vi "ICM aI8.vi"(11 "String In":string) -> (1 "Value I8":i8, 2 "Value":dbl, 3 "String Out":string)   [LabVIEW 2018]
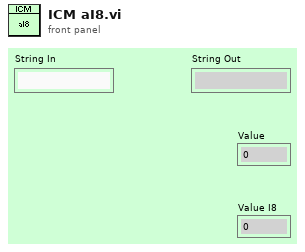
[diagram p1: front panel]
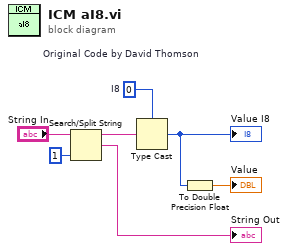
[diagram p0: block diagram]
diagram:
  w5 = i8 0  # I8
  n1 = Search/Split String(string="String In", offset (0)=1) -> (substring before match=w1:string, match + rest of string=→"String Out":string)  [unwired: 2 out]
  n2 = Type Cast "Original Code by David Thomson"(type=w5, x=w1) -> (*(type *) &x=w3:i8)
  "Value I8" <- w3
  n3 = To Double Precision Float(number=w3) -> (double precision float=→"Value":dbl)
